vi "VMUIStart_Viewer.vi"(6 "SetList VariableManager Ref in":refnum<vi>, 8 "error in (no error)":errorcluster, 10 "SubPanelRef":refnum<vi>, 11 "Viewer VariableManager Ref in":refnum<vi>) -> (0 "error out":errorcluster, 3 "Viewer VariableManagerRef out":refnum<vi>)   [LabVIEW 2013, in "VariableManagerAPI.lvlib"]
doc: "Start VariableManagerUserInterface. The user interface will be attached to the given sub panel reference.\n\nCreate a VariableManager object control in your application and give its referenct to this VI to start."
uses:
  VariableManagerAPI.lvlib
  VariableManager/VariableManager.lvclass
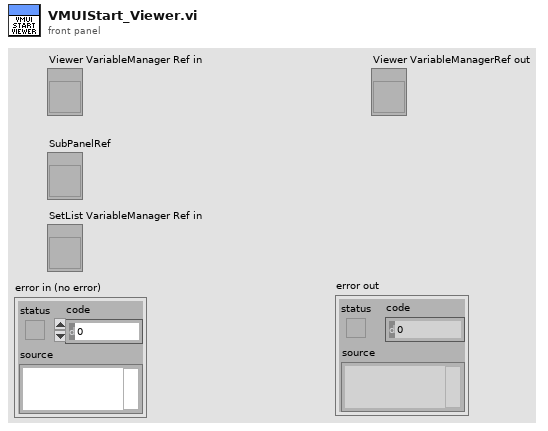
[diagram p1: front panel]
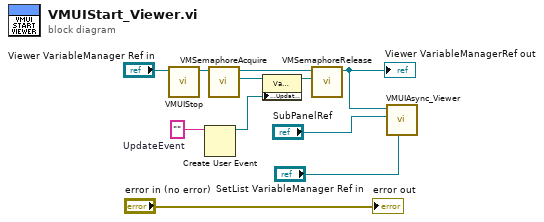
[diagram p0: block diagram]
diagram:
  w8 = ""  # UpdateEvent
  n1 = call "VMUIStop.vi"("VariableManagerRef in"="Viewer VariableManager Ref in") -> ("VariableManagerRef out"=w3:refnum<vi>)  [unwired: 9 in, 1 out]
  n2 = Create User Event(user event datatype=w8) -> (user event=w7:refnum<user-event>)  [unwired: 1 in, 1 out]
  n3 = call "VMSemaphoreAcquire.vi"("VariableManagerRef in"=w3) -> ("VariableManager"=w9:refnum<class "VariableManager.lvclass">, "VariableManagerRef out"=w10:refnum<vi>)  [unwired: 7 in, 2 out]
  n4 = property class="VariableManager.lvclass"(reference=w9, "Accessors:UpdateEvent"=w7) -> (reference out=w6:refnum<class "VariableManager.lvclass">)  [unwired: 1 in, 1 out]
  n5 = call "VMSemaphoreRelease.vi"("VariableManager"=w6, "VariableManagerRef in"=w10) -> ("VariableManagerRef out"=w5:refnum<vi>)  [unwired: 8 in, 1 out]
  "Viewer VariableManagerRef out" <- w5
  n6 = call "VMUIAsync_Viewer.vi"("SetList VariableManager ref"="SetList VariableManager Ref in", "SubPanelRef"="SubPanelRef", "VariableManagerRef in"=w5) -> ()  [unwired: 9 in]
  "error out" <- "error in (no error)"
